vi "TCP Stress Test.vi"() -> ()   [LabVIEW 2020]
uses:
  TCP Write.vi
panel:
  out "Graph":dbl[](graph)
  out "Sent":i32
  out "error out":errorcluster
  in  "Num writes":i32=100
  in  "IP Address":string="11.12.13.15"
  in  "Port":i32=4919
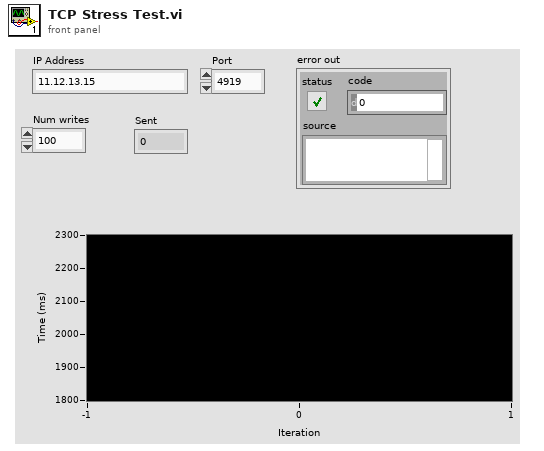
[diagram p1: front panel]
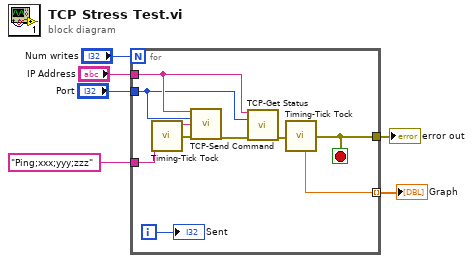
[diagram p0: block diagram]
diagram:
  n1 = for {
    N: "Num writes" -> [_]
    tunnel: "IP Address" -> [w9]
    tunnel: "Port" -> [w8]
    tunnel: "Ping;xxx;yyy;zzz" ("Command") -> [w15]
    tunnel: [w13] -> w2
    tunnel: [w11] -> w1 mode=indexing
    i -> [w12]
    stop <- w13 stop-if-true
    n2 = call "Timing-Tick Tock.vi"() -> ("error out"=w14:errorcluster)  [unwired: 6 in, 1 out]
    n3 = call "TCP-Send Command.vi"("PXI Address"=w9, "Port"=w8, "Command"=w15, "error in (no error)"=w14) -> ("error out"=w10:errorcluster)  [unwired: 11 in]
    n4 = call "TCP-Get Status.vi"("IP Address"=w9, "Port"=w8, "error in (no error)"=w10) -> ("error out"=w7:errorcluster)  [unwired: 11 in, 1 out]
    n5 = call "Timing-Tick Tock.vi"("error in (no error)"=w7) -> ("Elapsed time (ms)"=w11:dbl, "error out"=w13:errorcluster)  [unwired: 5 in]
    "Sent" <- w12
  }
  "error out" <- w2
  "Graph" <- w1
